vi "Convert All Files.vi"() -> ()   [LabVIEW 2023]
uses:
  <vilib>/SLL Drona/APIs/Stimulus/ControlValue/SetValueAuto.vi
  <vilib>/SLL Drona/Drona.lvlib
  <vilib>/SLL Drona/APIs/Stimulus/ControlValue/ControlValue.lvlib
panel:
  out "Numeric":i32
  out "Error Out":errorcluster
  in  "Error In":errorcluster
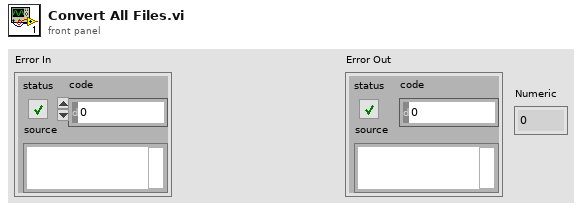
[diagram p1: front panel]
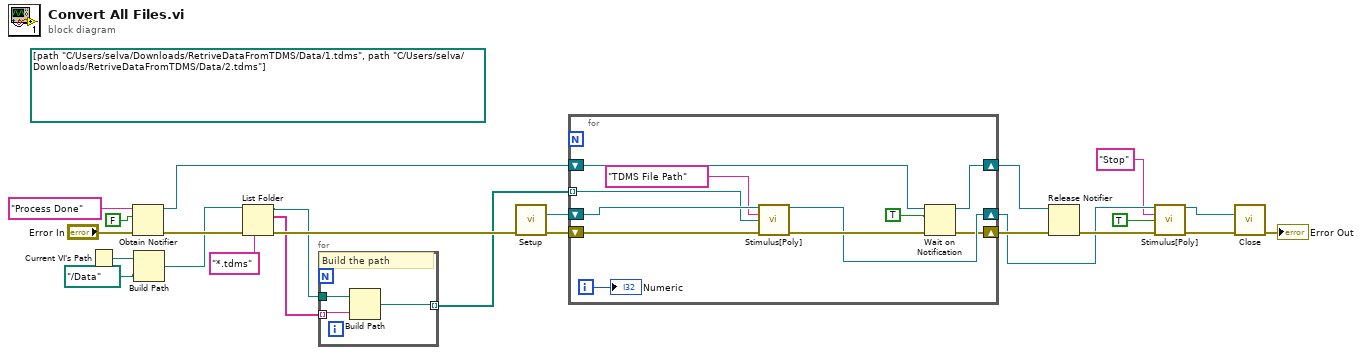
[diagram p0: block diagram]
diagram:
  (unwired) path[] [path "C:/Users/selva/Downloads/RetriveDataFromTDMS/Data/1.tdms", path "C:/Users/selva/Downloads/RetriveDataFromTDMS/Data/2.tdms"]
  n1 = Current VI's Path() -> (path=w12:path)
  n2 = Obtain Notifier(name (unnamed)="Process Done", notification data type=FALSE, error in (no error)="Error In") -> (notifier out=w17:refnum<notifier>, error out=w15:errorcluster)  [unwired: 1 in, 1 out]
  n3 = Build Path(base path=w12, name or relative path=path "../Data") -> (appended path=w10:path)
  n4 = List Folder(path=w10, pattern="*.tdms", error in=w15) -> (path out=w8:path, filenames=w9:string[], error out=w14:errorcluster)  [unwired: 1 in, 1 out]
  n5 = for {
    tunnel: w9 -> [w27] mode=indexing
    tunnel: w8 -> [w26]
    tunnel: [w25] -> w1 mode=indexing
    # "Build the path"
    n6 = Build Path(base path=w26, name or relative path=w27) -> (appended path=w25:path)
  }
  n7 = call <vilib>:"Setup.vi"("error in"=w14) -> ("VI Reference Out"=w22:refnum<vi>, "error out"=w23:errorcluster)  [unwired: 12 in, 1 out]
  n8 = for {
    tunnel: w1 -> [w35] mode=indexing
    shift-right: [w32] -> w18
    shift-left: w23 -> [w38]
    shift-right: [w33] -> w5
    shift-left: w22 -> [w37]
    shift-right: [w30] -> w16
    shift-left: w17 -> [w31]
    i -> [w28]
    n9 = call-poly <vilib>:"Stimulus[Poly].vi"("VI Reference In"=w37, "Control Path"="TDMS File Path", "Value (Signaling)"=w35, "error in"=w38) -> ("VI Reference Out"=w33:refnum<vi>, "error out"=w34:errorcluster)  [unwired: 10 in]
    n10 = Wait on Notification(notifier=w31, ignore previous (F)=TRUE, error in (no error)=w34) -> (notifier out=w30:refnum<notifier>, error out=w32:errorcluster)  [unwired: 1 in, 2 out]
    "Numeric" <- w28
  }
  n11 = Release Notifier(notifier=w16, error in (no error)=w18) -> (error out=w7:errorcluster)  [unwired: 1 in, 2 out]
  n12 = call-poly <vilib>:"Stimulus[Poly].vi"("VI Reference In"=w5, "Control Path"="Stop", "Value (Signaling)"=TRUE, "error in"=w7) -> ("VI Reference Out"=w2:refnum<vi>, "error out"=w6:errorcluster)  [unwired: 10 in]
  n13 = call <vilib>:"Close.vi"("VI Reference"=w2, "error in"=w6) -> ("error out"=→"Error Out":errorcluster)  [unwired: 13 in]
